vi "Phone Shift Notifier.vi"() -> ()   [LabVIEW 2014]
uses:
  <vilib>/smtpClient/Set Message Text.vi
  <vilib>/smtpClient/LabVIEWSMTPClient.lvlib
panel:
  in  "Password":string="fear4deer"
  in  "Email":string="kkleine4@gmail.com"
  in  "Message":string="This is a test."
  in  "Enum":enum16{"AT&T", "Sprint", "T-Mobile", "Verizon"}(ring)=enum."Verizon"
  in  "SMS Gateway":string[](array[string])=["@txt.att.net", "@messaging.sprintpcs.com", "@tmomail.net", "@vtext.com"]
  in  "Phone Number":string="9137070363"
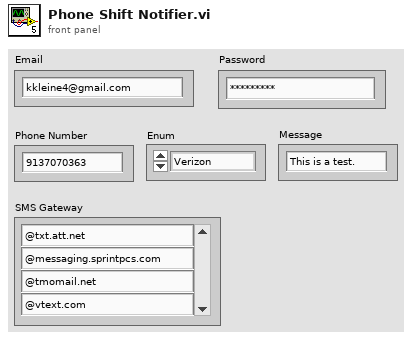
[diagram p1: front panel]
types:
  T1 = typedef "LabVIEWSMTPClient.lvlib/SmtpClientHandle.ctl" = refnum<k1>
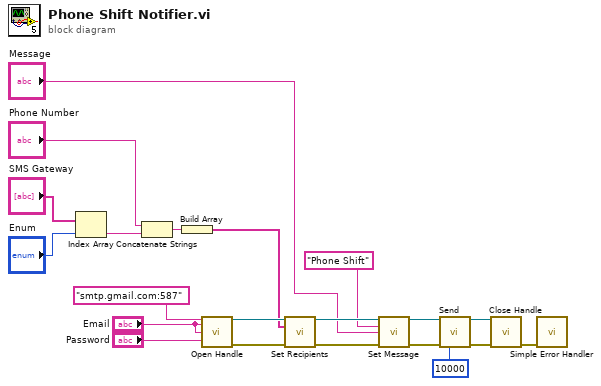
[diagram p0: block diagram]
diagram:
  n1 = Index Array(array="SMS Gateway", index="Enum") -> (element=w19:string)
  n2 = Concatenate Strings("Phone Number", w19) -> (w12:string)
  n3 = Build Array(w12) -> (w11:string[])
  n4 = call <vilib>:"Open Handle.vi"("server address"="smtp.gmail.com:587", "from"="Email", "username"="Email", "password"="Password") -> ("handle out"=w14:T1, "error out"=w13:errorcluster)  [unwired: 10 in]
  n5 = call <vilib>:"Set Recipients.vi"("handle in"=w14, "to"=w11, "error in (no error)"=w13) -> ("handle out"=w10:T1, "error out"=w9:errorcluster)  [unwired: 11 in]
  n6 = call-poly <vilib>:"Set Message.vi"("handle in"=w10, "subject"="Phone Shift", "plain text message"="Message", "error in (no error)"=w9) -> ("handle out"=w6:T1, "error out"=w5:errorcluster)  [unwired: 10 in]
  n7 = call <vilib>:"Send.vi"("handle in"=w6, "error in (no error)"=w5, "timeout in ms (10000)"=10000) -> ("handle out"=w3:T1, "error out"=w2:errorcluster)  [unwired: 10 in, 1 out]
  n8 = call <vilib>:"Close Handle.vi"("handle in"=w3, "error in (no error)"=w2) -> ("error out"=w1:errorcluster)  [unwired: 12 in, 1 out]
  n9 = call <vilib>:"Simple Error Handler.vi"("error in (no error)"=w1) -> ()  [unwired: 4 in, 5 out]
